vi "DoesScriptNumberContainNull.vi"(10 "Script Index":i32) -> (1 "Contains Null?":bool)   [LabVIEW 2015]
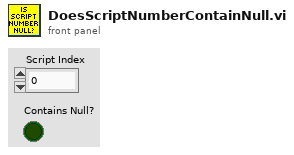
[diagram p1: front panel]
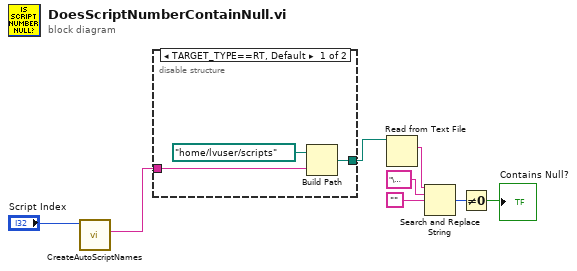
[diagram p0: block diagram]
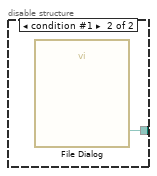
[diagram p2: hidden frame]
diagram:
  n1 = call "CreateAutoScriptNames.vi"("Index"="Script Index") -> ("Concat String"=w2:string)  [unwired: 10 in]
  n2 = disable-structure shown="TARGET_TYPE==RT, Default" {
    disable-tunnel: w2 -> [w11 _]
    disable-tunnel: [w9 w12] -> w5
    frame condition #0 (active) {
      n3 = Build Path(base path=path "/home/lvuser/scripts", name or relative path=w11) -> (appended path=w9:path)
    }
    frame condition #1 {
      n4 = call "File Dialog"() -> ("selected path"=w12:path)  [unwired: 7 in, 8 out]
    }
  }
  n5 = Read from Text File(file (use dialog)=w5) -> (text=w4:string)  [unwired: 1 in, 5 out]
  n6 = Search and Replace String(input string=w4, search string="\u0000" ("regular expression"), replace string="") -> (number of replacements=w6:i32)  [unwired: 5 in, 3 out]
  n7 = Not Equal To 0?(x=w6) -> (x != 0?=→"Contains Null?":bool)
